vi "Shifter.vi"(8 "error in (no error)":errorcluster, 10 "Solenoid On?":bool, 11 "DoubleSolenoid in":refnum<class "DoubleSolenoid.lvclass">) -> (0 "error out":errorcluster, 3 "DoubleSolenoid out":refnum<class "DoubleSolenoid.lvclass">)   [LabVIEW 2018, in "Pneumatics control.lvlib" / "DoubleSolenoid.lvclass"]
doc: "This VI switches the pneumatic piston from HIGH to LOW depending on the boolean that arrives. If the boolean does not change, and the switching time has elapsed, then it will keep the solenid off."
uses:
  DoubleSolenoid.lvclass
  C:/Users/Public/Documents/2019DeepSpace/Classes/Pnematics control/Solenoids/Solenoids.lvclass
  DoubleSolenoid.lvclass/DoubleSolenoid.ctl
  <vilib>/Rock Robotics/WPI/Solenoid/WPI_SolenoidValue.ctl
  <vilib>/Rock Robotics/WPI/Solenoid/WPI_SolenoidSetEnum.vi
  Solenoids.lvclass
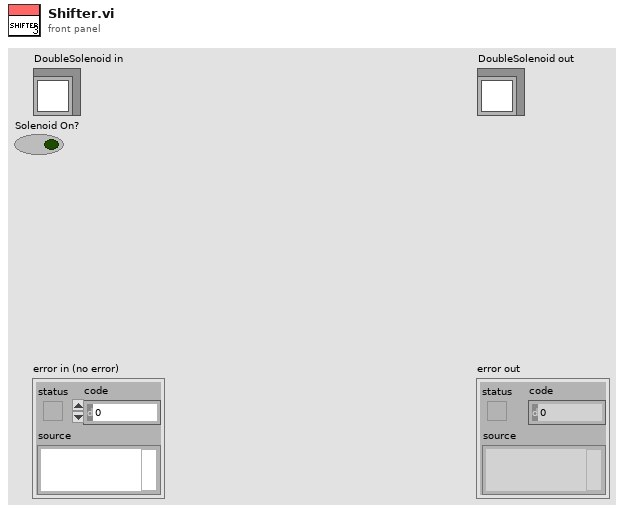
[diagram p1: front panel]
types:
  T1 = typedef "WPI_SolenoidValue.ctl" = enum16{"Off", "On", "Forward", "Reverse"}
  T2 = typedef "WPI_SolenoidDevRef.ctl" = cluster{"DevStatus":errorcluster, "Pneumatics Control Module":u8, "Forward Solenoid Channel":T3, "Reverse Solenoid Channel":T3}
  T3 = typedef "WPI_SolenoidChannel.ctl" = enum8{"Solenoid 0", "Solenoid 1", "Solenoid 2", "Solenoid 3", "Solenoid 4", "Solenoid 5", "Solenoid 6", "Solenoid 7", "Invalid"}
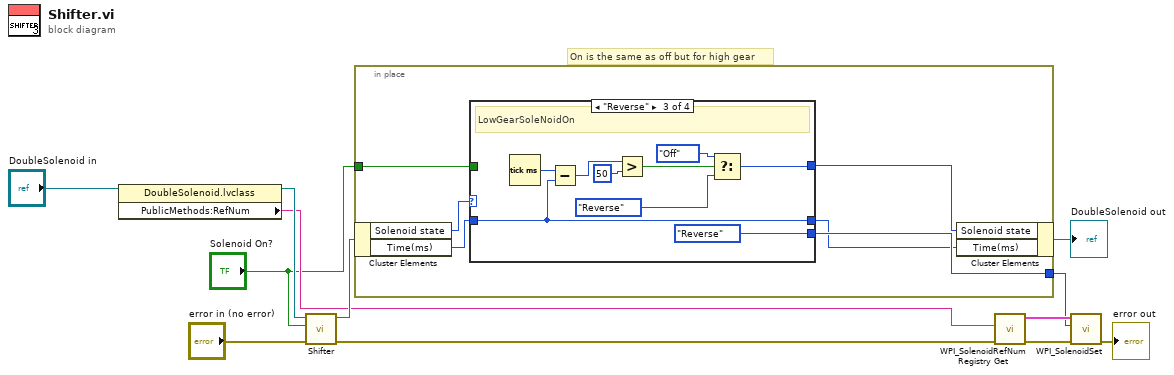
[diagram p0: block diagram]
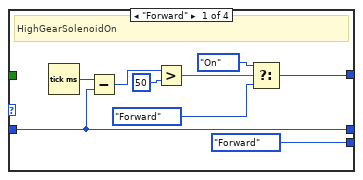
[diagram p2: hidden frame]
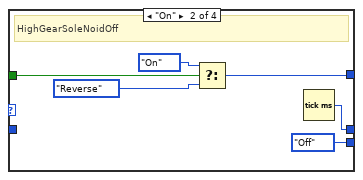
[diagram p3: hidden frame]
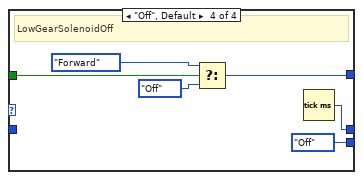
[diagram p4: hidden frame]
diagram:
  # "On is the same as off but for high gear"
  n1 = property class="DoubleSolenoid.lvclass"(reference="DoubleSolenoid in") -> (reference out=w7:refnum<class "DoubleSolenoid.lvclass">, "PublicMethods:RefNum"=w6:string)  [unwired: 1 in, 1 out]
  n2 = call-parent "Shifter.vi"("error in (no error)"="error in (no error)", "Solenoid On?"="Solenoid On?", "Solenoids in"=w7) -> ("error out"=w2:errorcluster, "Solenoids out"=w10:refnum<class "DoubleSolenoid.lvclass">)  [unwired: 7 in]
  n3 = in-place {
    in-place-border: "Solenoid On?" -> [w17]
    in-place-border: [w16] -> w4
    n4 = in-place-cluster #1(w10) -> ("Solenoid state"=w18:T1, "Time(ms)"=w13:u32)
    n5 = case shown="\"Reverse\"" w18 {
      tunnel: w17 -> [_ w31 _ w48]
      tunnel: [WPI_SolenoidValue."Forward" ("Value") WPI_SolenoidValue."Off" ("Value") WPI_SolenoidValue."Reverse" ("Value") WPI_SolenoidValue."Off" ("Value")] -> w16
      tunnel: [w20 w28 w35 w44] -> w15
      tunnel: [w19 w32 w34 w43] -> w14
      tunnel: w13 -> [w19 _ w34 _]
      frame "Forward" {
        # "HighGearSolenoidOn"
        n6 = Tick Count (ms)() -> (millisecond timer value=w24:u32)
        n7 = Subtract(x=w24, y=w19) -> (x-y=w23:u32)
        n8 = Greater?(x=w23, y=u32 50) -> (0:w21:bool)
        n9 = Select(t=WPI_SolenoidValue."On" ("Solenoid state"), s=w21, f=WPI_SolenoidValue."Forward" ("Solenoid state")) -> (s? t:f=w20:T1)
      }
      frame "On" {
        # "HighGearSoleNoidOff"
        n10 = Select(t=WPI_SolenoidValue."On" ("Value"), s=w31, f=WPI_SolenoidValue."Reverse" ("Value")) -> (s? t:f=w28:T1)
        n11 = Tick Count (ms)() -> (millisecond timer value=w32:u32)
      }
      frame "Reverse" {
        # "LowGearSoleNoidOn"
        n12 = Tick Count (ms)() -> (millisecond timer value=w40:u32)
        n13 = Subtract(x=w40, y=w34) -> (x-y=w39:u32)
        n14 = Greater?(x=w39, y=u32 50) -> (0:w37:bool)
        n15 = Select(t=WPI_SolenoidValue."Off" ("Solenoid state"), s=w37, f=WPI_SolenoidValue."Reverse" ("Solenoid state")) -> (s? t:f=w35:T1)
      }
      frame "Off", Default {
        # "LowGearSolenoidOff"
        n16 = Select(t=WPI_SolenoidValue."Forward" ("Solenoid state"), s=w48, f=WPI_SolenoidValue."Off" ("Solenoid state")) -> (s? t:f=w44:T1)
        n17 = Tick Count (ms)() -> (millisecond timer value=w43:u32)
      }
    }
    n18 = in-place-cluster #1("Solenoid state"=w15, "Time(ms)"=w14) -> (→"DoubleSolenoid out":refnum<class "DoubleSolenoid.lvclass">)
  }
  n19 = call <vilib>:"WPI_SolenoidRefNum Registry Get.vi"("error in (no error)"=w2, "refnum name"=w6) -> ("error out"=w5:errorcluster, "SolenoidDevRef"=w8:T2)  [unwired: 8 in]
  n20 = call-poly <vilib>:"WPI_SolenoidSet.vi"("error in (no error)"=w5, "Value"=w4, "SolenoidDevRef"=w8) -> ("error out"=→"error out":errorcluster)  [unwired: 7 in, 1 out]
